vi "Air Loop.vi"(6 "Louver Position (% Open)":dbl, 8 "input cluster":T1, 9 "Air Inlet Temperature (K)":dbl, 10 "NDHX Heat Transfer (W)":dbl, 11 "Time Interval (s)":dbl) -> (0 "Indications":dbl[](array[numeric]), 1 "Heat Rejection (W)":dbl, 2 "Air Average Viscosity (Pa-s)":dbl, 3 "Air Outlet Temperature (K)":dbl)   [LabVIEW 2019]
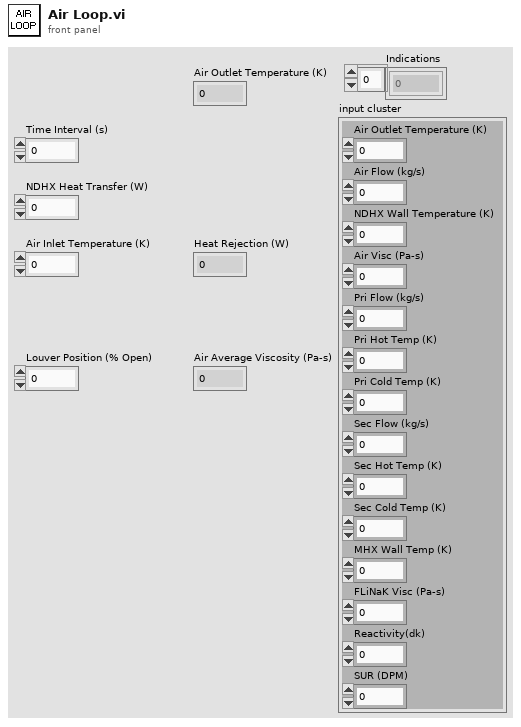
[diagram p1: front panel]
types:
  T1 = cluster{"Air Outlet Temperature (K)":dbl, "Air Flow (kg/s)":dbl, "NDHX Wall Temperature (K)":dbl, "Air Visc (Pa-s)":dbl, "Pri Flow (kg/s)":dbl, "Pri Hot Temp (K)":dbl, "Pri Cold Temp (K)":dbl, "Sec Flow (kg/s)":dbl, "Sec Hot Temp (K)":dbl, "Sec Cold Temp (K)":dbl, "MHX Wall Temp (K)":dbl, "FLiNaK Visc (Pa-s)":dbl, "Reactivity(dk)":dbl, "SUR (DPM)":dbl}
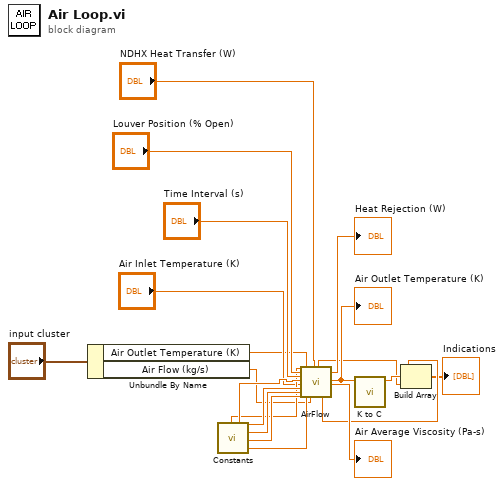
[diagram p0: block diagram]
diagram:
  n1 = Unbundle By Name("input cluster") -> ("Air Outlet Temperature (K)"=w2:dbl, "Air Flow (kg/s)"=w3:dbl)
  n2 = call "Constants.vi"() -> ("Stack Height (m)"=w9:dbl, "NDHX Tube Pitch (m)"=w10:dbl, "NDHX Tube Diameter (m)"=w11:dbl, "NDHX Tube Length (m)"=w12:dbl, "Stack Inner Diameter"=w13:dbl, "NDHX Number of Tubes"=w14:dbl)  [unwired: 5 in, 17 out]
  n3 = call "AirFlow.vi"("Stack Height (m)"=w9, "Louver Position (% Open)"="Louver Position (% Open)", "Time Interval (s)"="Time Interval (s)", "NDHX Tube Pitch (m)"=w10, "Air Cold Temperature (K)"="Air Inlet Temperature (K)", "NDHX Tube Diameter (m)"=w11, "NDHX Tube Length (m)"=w12, "Stack Inner Diameter (m)"=w13, "Air Hot Temperature (K)"=w2, "NDHX Number of Tubes"=w14, "Air Mass Flow (kg/s)"=w3, "NDHX Heat Transfer (W)"="NDHX Heat Transfer (W)") -> ("Air Ave Temperature (C)"=w5:dbl, "Air Mass Flow (kg/s)"=w7:dbl, "Heat Rejection (W)"=→"Heat Rejection (W)":dbl, "Air Outlet Temperature (K)"=w18:dbl, "Air Average Viscosity (Pa-s)"=→"Air Average Viscosity (Pa-s)":dbl)  [unwired: 1 in, 10 out]
  "Air Outlet Temperature (K)" <- w18
  n4 = call "K to C.vi"("Temperature (K)"=w18) -> ("Temperature (C)"=w6:dbl)  [unwired: 10 in]
  n5 = Build Array(w7, w6, w5) -> (→"Indications":dbl[])
